vi "VariablesToString_Array.vi"(1 "Terminate?":bool=TRUE, 2 "ValueIn":dbl[](array[numeric]), 3 "KeyWord":string) -> (0 "StringOut":string)   [LabVIEW 2011]
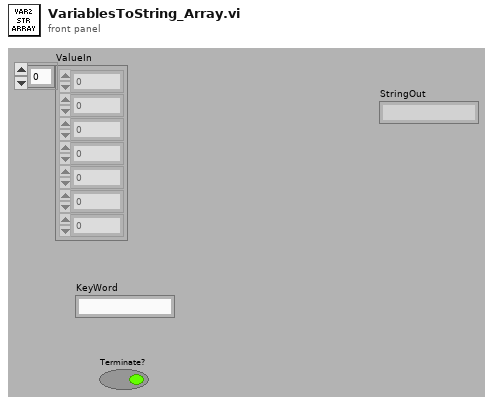
[diagram p1: front panel]
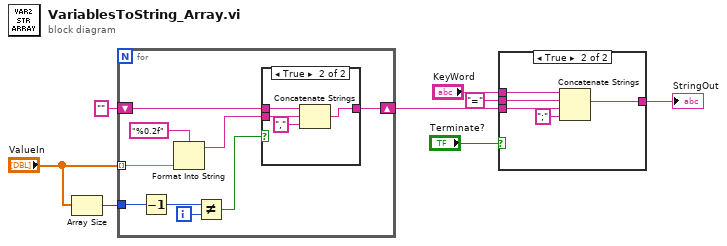
[diagram p0: block diagram]
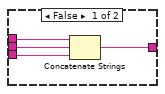
[diagram p2: hidden frame]
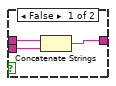
[diagram p3: hidden frame]
diagram:
  n1 = Array Size(array="ValueIn") -> (size(s)=w8:i32)
  n2 = for {
    tunnel: "ValueIn" -> [w17] mode=indexing
    shift-right: [w15] -> w3
    shift-left: "" -> [w14]
    tunnel: w8 -> [w12]
    i -> [w10]
    n3 = Decrement(x=w12) -> (x-1=w11:i32)
    n4 = Format Into String(format string="%0.2f", w17) -> (resulting string=w13:string)  [unwired: 2 in, 1 out]
    n5 = Not Equal?(x=w11, y=w10) -> (x != y?=w9:bool)
    n6 = case shown="True" w9 {
      tunnel: [w18 w24] -> w15
      tunnel: w14 -> [w20 w23]
      tunnel: w13 -> [w19 w22]
      frame False {
        n7 = Concatenate Strings(w20, w19) -> (w18:string)
      }
      frame True {
        n8 = Concatenate Strings(w23, w22, "," ("string")) -> (w24:string)
      }
    }
  }
  n9 = case shown="True" "Terminate?" {
    tunnel: "KeyWord" -> [w28 w33]
    tunnel: "=" ("string") -> [w27 w32]
    tunnel: w3 -> [w26 w31]
    tunnel: [w25 w29] -> w1
    frame False {
      n10 = Concatenate Strings(w28, w27, w26) -> (w25:string)
    }
    frame True {
      n11 = Concatenate Strings(w33, w32, w31, ";" ("string")) -> (w29:string)
    }
  }
  "StringOut" <- w1
